vi "Close.vi"(8 "error in (no error)":errorcluster, 11 "Hitec HS400 Series in":refnum<class "Hitec HS400 Series.lvclass">) -> (0 "error out":errorcluster)   [LabVIEW 2013, in "Hitec HS400 Series.lvclass"]
doc: "Terminates the software connection to the sensor."
uses:
  Hitec HS400 Series.lvclass
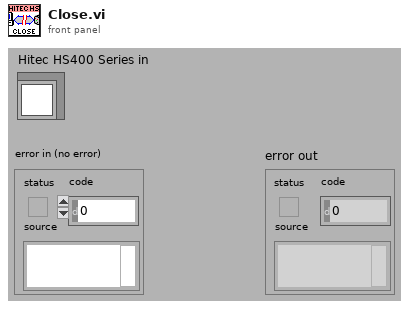
[diagram p1: front panel]
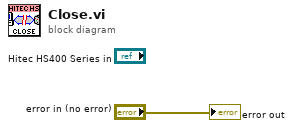
[diagram p0: block diagram]
diagram:
  "error out" <- "error in (no error)"
